vi "항법좌표계 변환.vi"(2 "Y_TM":dbl format="%#.8g", 3 "X_TM":dbl format="%#.8g") -> (0 "Y_Nav":dbl format="%#.8g", 1 "X_Nav":dbl format="%#.8g")   [LabVIEW 2016]
uses:
  <vilib>/imath/engines/lvmath2/RunTimeEngine/Managers/WorkSpace/UID Generator.vi
  <vilib>/imath/engines/lvmath2/RunTimeEngine/RunTimeType/NIMS_RunTimeType_From StrictType (excl LVString).vi
  <instcachedir>/0/NIMS_RunTimeType_From StrictType (excl LVString)_BBF44FB49F834B71AF7A14CCEDF8BECD.lvgen/NIMS_RunTimeType_From StrictType (excl LVString)_BBF44FB49F834B71AF7A14CCEDF8BECD_000.vi
  <vilib>/imath/engines/lvmath2/RunTimeEngine/LocalVariableDefStatement/MC_LocalVariableDefStatement_Display.vi
  <vilib>/imath/engines/lvmath2/RunTimeEngine/Managers/SymbolTable/Clear UID.vi
  <vilib>/imath/engines/lvmath2/RunTimeEngine/NodeEndStatement/NIMS_NodeEndStatement_Output.vi
  <instcachedir>/0/NIMS_NodeEndStatement_Output_53EC0D466D134D7ABD903AC30B43404B.lvgen/NIMS_NodeEndStatement_Output_53EC0D466D134D7ABD903AC30B43404B_001.vi
  <vilib>/imath/engines/lvmath2/RunTimeEngine/ErrorHandling/NIMS_Finalize Error.vi
  <vilib>/imath/engines/lvmath2/RunTimeEngine/Managers/SymbolTable/NIMS_WorkSpace.lvlib
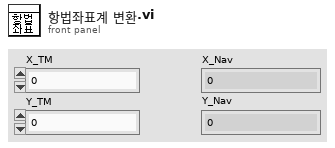
[diagram p1: front panel]
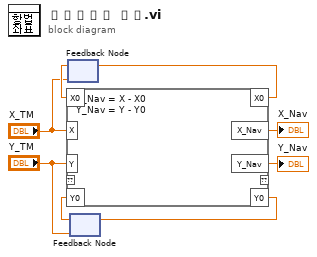
[diagram p0: block diagram]
diagram:
  n1 = feedback #1("X_TM") -> (w7:dbl)
  n2 = feedback #2("Y_TM") -> (w5:dbl)
  n3 = mathscript code="X_Nav = X - X0\nY_Nav = Y - Y0"("X0"=w7, "Y0"=w5, "X"="X_TM", "Y"="Y_TM") -> ("X0"=w8:dbl, "Y0"=w6:dbl, "X_Nav"=→"X_Nav":dbl, "Y_Nav"=→"Y_Nav":dbl)  [unwired: 1 in, 1 out]
  n4 = feedback-in #1(w8) -> ()
  n5 = feedback-in #2(w6) -> ()
